vi "Ciclo_while_max_min_contador_promedio.vi"() -> ()   [LabVIEW 2013]
panel:
  out "contador":dbl
  out "Menor":dbl
  out "Mayor":dbl
  out "Promedio":dbl
  out "Temperatura":i32(slide) scale=0.0..60.0
  # "Generar 10 temperaturas , y al final presentar la temperatura mayor , menor y la temperatura promedio"
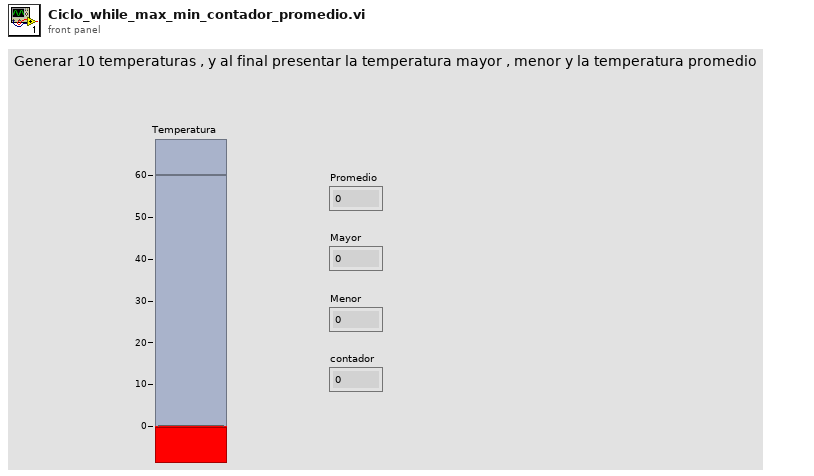
[diagram p1: front panel]
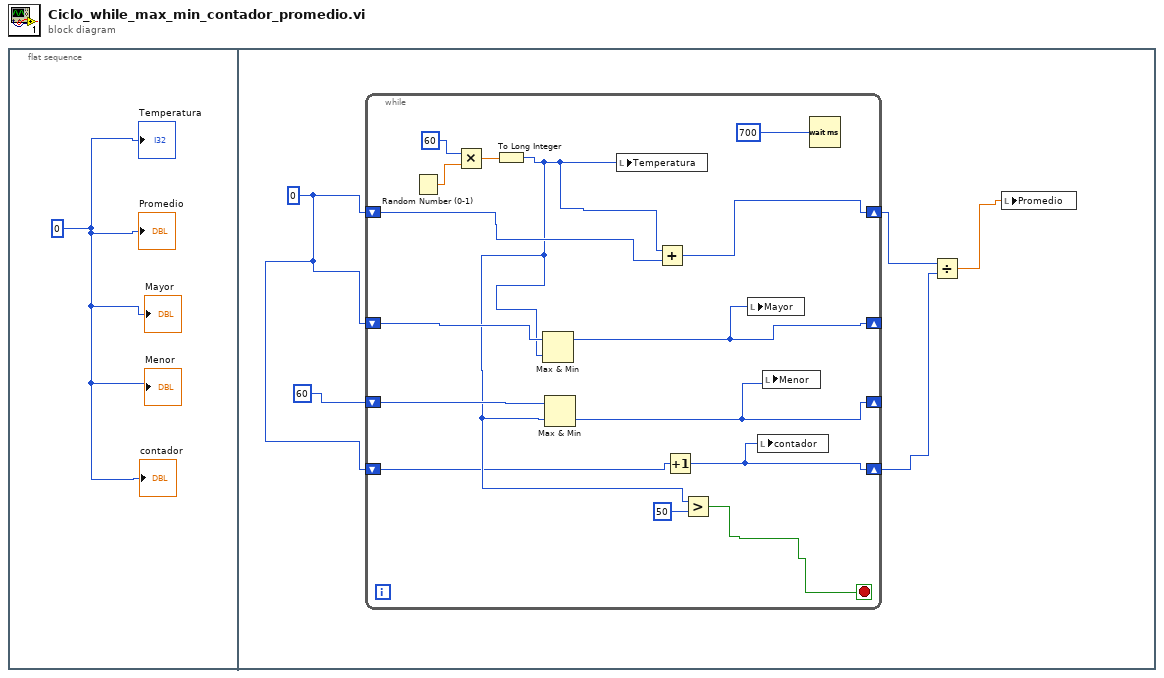
[diagram p0: block diagram]
diagram:
  n1 = flat-sequence {
    frame #0 {
      w1 = 0
      "Temperatura" <- w1
      "Promedio" <- w1
      "Mayor" <- w1
      "Menor" <- w1
      "contador" <- w1
    }
    frame #1 {
      w3 = 0
      n2 = while {
        shift-right: [w17] -> w6
        shift-left: w3 -> [w18]
        shift-right: [w13] -> _
        shift-left: w3 -> [w15]
        shift-right: [w12] -> _
        shift-left: 60 -> [w14]
        shift-right: [w7] -> w2
        shift-left: w3 -> [w8]
        stop <- w11 stop-if-true
        n3 = Random Number (0-1)() -> (number: 0 to 1=w21:dbl)
        n4 = Multiply(x=60, y=w21) -> (x*y=w19:dbl)
        n5 = To Long Integer(number=w19) -> (32bit integer=w10:i32)
        n6 = Max & Min(x=w15, y=w10) -> (max(x,y)=w13:i32)  [unwired: 1 out]
        n7 = Max & Min(x=w14, y=w10) -> (min(x,y)=w12:i32)  [unwired: 1 out]
        n8 = local write "Temperatura"(w10) -> ()
        n9 = Add(x=w10, y=w18) -> (x+y=w17:i32)
        n10 = Increment(x=w8) -> (x+1=w7:i32)
        n11 = Greater?(x=w10, y=50) -> (0:w11:bool)
        n12 = local write "Mayor"(w13) -> ()
        n13 = local write "contador"(w7) -> ()
        n14 = local write "Menor"(w12) -> ()
        n15 = Wait (ms)(milliseconds to wait=700) -> ()  [unwired: 1 out]
      }
      n16 = Divide(x=w6, y=w2) -> (x/y=w5:dbl)
      n17 = local write "Promedio"(w5) -> ()
    }
  }
